vi "Write Positions to File.vi"(8 "error in (no error)":errorcluster, 11 "positions":T1[](array[typedef])) -> (0 "error out":errorcluster)   [LabVIEW 2020, in "Manipulator.lvlib"]
uses:
  Manipulator.lvlib
  Named Position.ctl
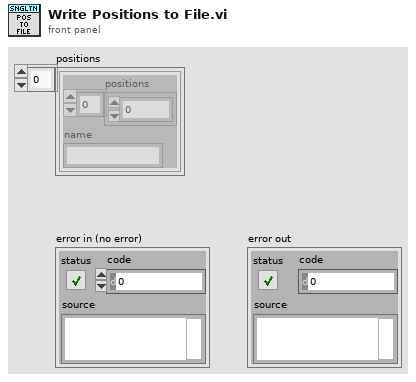
[diagram p1: front panel]
types:
  T1 = typedef "Manipulator.lvlib/Named Position.ctl" = cluster{"positions":dbl[], "name":string}
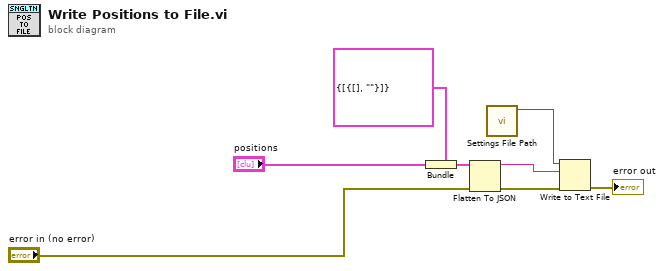
[diagram p0: block diagram]
diagram:
  n1 = Bundle(cluster=cluster{"named_positions":T1[]} {"named_positions"=[{"positions"=[], "name"=""}]}, "named_positions"="positions") -> (w7:cluster{"named_positions":T1[]})
  n2 = Flatten To JSON(anything=w7, error in (no error)="error in (no error)") -> (JSON string=w2:string, 11:w3:errorcluster)  [unwired: 1 in]
  n3 = call "Settings File Path.vi"() -> ("settings path"=w4:path)  [unwired: 11 in]
  n4 = Write to Text File(file (use dialog)=w4, text=w2, error in=w3) -> (error out=→"error out":errorcluster)  [unwired: 1 in, 2 out]
